vi "CS POLARIS BME DG.destructor.vi"(0 "i ref in":refnum<vi>, 5 "error in (no error)":errorcluster) -> (19 "error out":errorcluster)   [LabVIEW 2009, in "CS POLARIS BME DG.lvlib"]
doc: "This is the destructor of a class.\n\nLicense Agreement for this software:\n\nCopyright (C)\nGesellschaft für Schwerionenforschung, GSI\nPlanckstr. 1\n64291 Darmstadt\nGermany\n\nContact: D.Beck@gsi.de \n\nThis program is free software; you can redistribute it and/or modify it under the terms of the \nGNU General Public License as published by the Free Software Foundation; either version 2 of \nthe license, or (at your option) any later version.\n\nThis program is distributed in the hope that it will be useful, but WITHOUT ANY WARRANTY; \nwithout even the implied warranty of MERCHANTABILITY or FITNESS FOR A PARTICULAR PURPOSE. See the GNU General License for more details (http://www.gnu.org).\n\nGesellschaft für Schwerionenforschung, GSI\nPlanckstr. 1, 64291 Darmstadt, Germany\nFor all questions and ideas contact: M.Richter@gsi.de, H.Brand@gsi.de or D.Beck@gsi.de.\nLast update: 16-JUN-2004"
uses:
  CS POLARIS BME DG.lvlib
  CSApplicationBaseClasses/DeviceBase/DeviceBase.lvlib
  DG Classes/BME_DG_System/BME_DG_System.lvclass
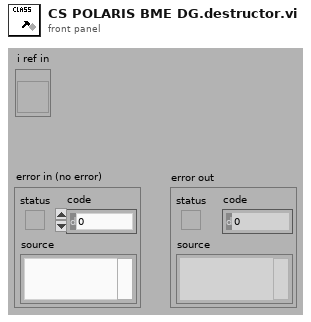
[diagram p1: front panel]
types:
  T1 = enum16{"SetAttribute", "GetAttribute", "CreateAttribute", "DestroyAttribute", "DestroyAllAtributes"}
  T2 = typedef "CS POLARIS BME DG.lvlib/CS POLARIS BME DG.i attribute.ctl" = cluster{"Numeric":dbl, "DG_System":refnum<queue>, "UpdateTasks":refnum<queue>}
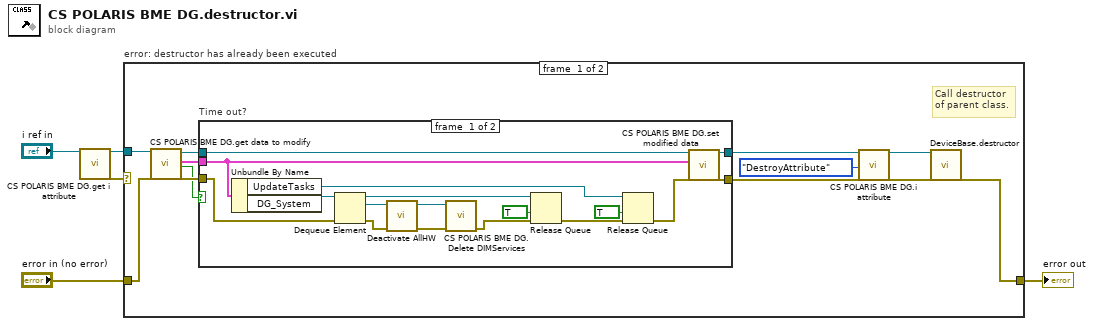
[diagram p0: block diagram]
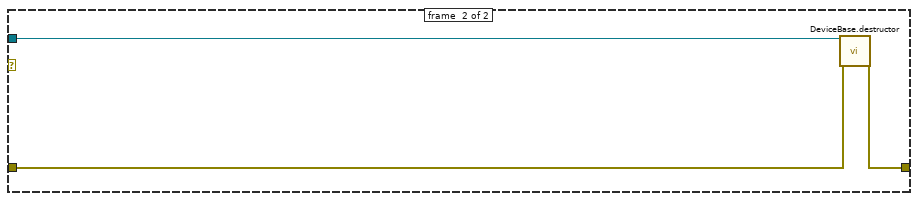
[diagram p3: hidden frame]
diagram:
  n1 = call "CS POLARIS BME DG.get i attribute.vi"("i ref in"="i ref in") -> ("i ref out"=w1:refnum<vi>, "error out"=w2:errorcluster)  [unwired: 16 in, 1 out]
  n2 = case "error: destructor has already been executed" shown="No Error" w2 {
    tunnel: [w14 w38] -> w5
    tunnel: "error in (no error)" -> [w9 w39]
    tunnel: w1 -> [w12 w37]
    frame #0 {
      # "Call destructor\nof parent class."
      n3 = call "CS POLARIS BME DG.get data to modify.vi"("i ref in"=w12, "error in (no error)"=w9) -> ("i ref out"=w13:refnum<vi>, "i attribute"=w6:T2, "timed out"=w7:bool, "error out"=w10:errorcluster)  [unwired: 14 in]
      n4 = case "Time out?" shown="False" w7 {
        tunnel: w13 -> [w34 w36]
        tunnel: [w33 w36] -> w11
        tunnel: w10 -> [w26 w35]
        tunnel: [w32 w35] -> w8
        tunnel: w6 -> [w31 _]
        frame #0 {
          n5 = Unbundle By Name(w31) -> ("UpdateTasks"=w23:refnum<queue>, "DG_System"=w28:refnum<queue>)
          n6 = Dequeue Element(queue=w28, error in (no error)=w26) -> (queue out=w27:refnum<queue>, element=w25:refnum<class "BME_DG_System.lvclass">, error out=w24:errorcluster)  [unwired: 1 in, 1 out]
          n7 = call "Deactivate AllHW.vi"("error in (no error)"=w24, "BME_DG_System in"=w25) -> ("error out"=w21:errorcluster, "BME_DG_System out"=w22:refnum<class "BME_DG_System.lvclass">)  [unwired: 8 in]
          n8 = call "CS POLARIS BME DG.Delete DIMServices.vi"("error in (no error)"=w21, "BME_DG_System in"=w22) -> ("error out"=w20:errorcluster)  [unwired: 8 in, 1 out]
          n9 = Release Queue(queue=w27, force destroy? (F)=TRUE, error in (no error)=w20) -> (error out=w30:errorcluster)  [unwired: 2 out]
          n10 = Release Queue(queue=w23, force destroy? (F)=TRUE, error in (no error)=w30) -> (error out=w29:errorcluster)  [unwired: 2 out]
          n11 = call "CS POLARIS BME DG.set modified data.vi"("i ref in"=w34, "i attribute"=w31, "error in (no error)"=w29) -> ("i ref out"=w33:refnum<vi>, "error out"=w32:errorcluster)  [unwired: 15 in]
        }
        frame #1 {
        }
      }
      n12 = call "CS POLARIS BME DG.i attribute.vi"("VI Refnum"=w11, "Action"=T1."DestroyAttribute", "error in (no error)"=w8) -> ("VI Refnum out"=w16:refnum<vi>, "error out"=w15:errorcluster)  [unwired: 14 in, 1 out]
      n13 = call "DeviceBase.destructor.vi"("i ref in"=w16, "error in (no error)"=w15) -> ("error out"=w14:errorcluster)  [unwired: 17 in]
    }
    frame #1 {
      n14 = call "DeviceBase.destructor.vi"("i ref in"=w37, "error in (no error)"=w39) -> ("error out"=w38:errorcluster)  [unwired: 17 in]
    }
  }
  "error out" <- w5
